vi "DSP_RegisterWrite.vi"(2 "error in (no error)":errorcluster, 3 "Value":u32, 4 "Offset":u32, 5 "Board Handle":u64) -> (0 "error out":errorcluster, 1 "Board Handle Out":u64)   [LabVIEW 2009]
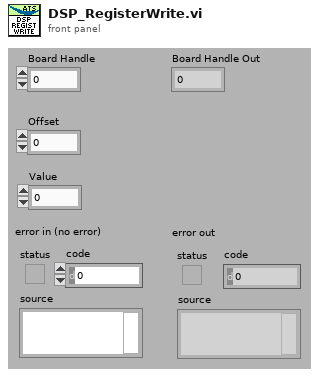
[diagram p1: front panel]
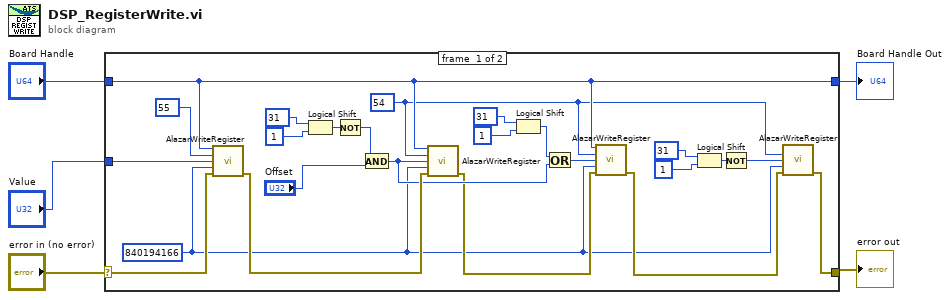
[diagram p0: block diagram]
diagram:
  n1 = case shown="No Error" "error in (no error)" {
    selector: "error in (no error)" -> [w29 w31]
    tunnel: [w6 w31] -> w4
    tunnel: [w16 w30] -> w3
    tunnel: "Board Handle" -> [w16 w30]
    tunnel: "Value" -> [w27 _]
    frame #0 {
      w12 = u32 54
      w10 = u32 840194166
      n2 = call "AlazarWriteRegister.vi"("Board Handle"=w16, "Offset"=u32 55, "Value"=w27, "Password"=w10, "error in (no error)"=w29) -> ("error out"=w21:errorcluster)  [unwired: 8 in, 2 out]
      n3 = Logical Shift(y=31, x=u32 1) -> (x << y=w24:u32)
      n4 = Not(x=w24) -> (.not. x?=w23:u32)
      n5 = And(x=w23, y="Offset") -> (x .and. y?=w17:u32)
      n6 = call "AlazarWriteRegister.vi"("Board Handle"=w16, "Offset"=w12, "Value"=w17, "Password"=w10, "error in (no error)"=w21) -> ("error out"=w15:errorcluster)  [unwired: 8 in, 2 out]
      n7 = Logical Shift(y=31, x=u32 1) -> (x << y=w18:u32)
      n8 = Or(x=w18, y=w17) -> (x .or. y?=w9:u32)
      n9 = call "AlazarWriteRegister.vi"("Board Handle"=w16, "Offset"=w12, "Value"=w9, "Password"=w10, "error in (no error)"=w15) -> ("error out"=w11:errorcluster)  [unwired: 8 in, 2 out]
      n10 = Logical Shift(y=31, x=u32 1) -> (x << y=w8:u32)
      n11 = Not(x=w8) -> (.not. x?=w7:u32)
      n12 = call "AlazarWriteRegister.vi"("Offset"=w12, "Value"=w7, "Password"=w10, "error in (no error)"=w11) -> ("error out"=w6:errorcluster)  [unwired: 9 in, 2 out]
    }
    frame #1 {
    }
  }
  "Board Handle Out" <- w3
  "error out" <- w4
